vi "0-Write MDF.vi"(3 "List of Waypoints":T1 {"Waypoints Array"."Point Type" items=["Drive", "Round Port", "Round Starboard", "Stay"]}) -> ()   [LabVIEW 2011]
uses:
  0x2-OCU-Think Comm/0x2 Typedefs/ocuWaypoints.ctl
  0x2-OCU-Think Comm/0x2 Typedefs/ocuWaypoint.ctl
  0x2-OCU-Think Comm/0x2 Typedefs/waypointTypes.ctl
  2-Think/2 Typedefs/UTM Location.ctl
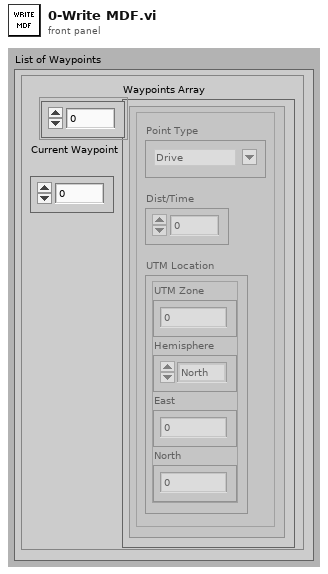
[diagram p1: front panel]
types:
  T1 = typedef "ocuWaypoints.ctl" = cluster{"Waypoints Array":T2[], "Current Waypoint":dbl}
  T2 = typedef "ocuWaypoint.ctl" = cluster{"Point Type":T3, "Dist/Time":dbl, "UTM Location":T4}
  T3 = typedef "waypointTypes.ctl" = u16
  T4 = typedef "UTM Location.ctl" = cluster{"UTM Zone":dbl, "Hemisphere":enum16{"North", "South"}, "East":dbl, "North":dbl}
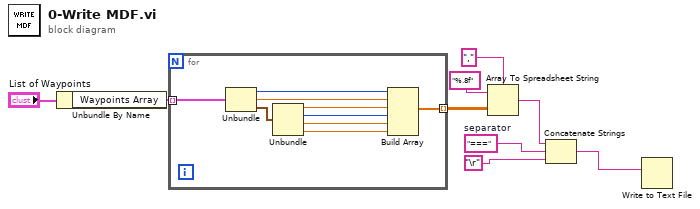
[diagram p0: block diagram]
diagram:
  w5 = "==="  # separator
  n1 = Unbundle By Name("List of Waypoints") -> ("Waypoints Array"=w2:T2[])
  n2 = for {
    tunnel: w2 -> [w18] mode=indexing
    tunnel: [w10] -> w1 mode=indexing
    n3 = Unbundle(w18) -> ("Point Type"=w16:T3, "Dist/Time"=w15:dbl, "UTM Location"=w17:T4)
    n4 = Unbundle(w17) -> ("UTM Zone"=w14:dbl, "Hemisphere"=w13:enum16{"North", "South"}, "East"=w12:dbl, "North"=w11:dbl)
    n5 = Build Array(w16, w15, w14, w13, w12, w11) -> (w10:dbl[])
  }
  n6 = Array To Spreadsheet String(delimiter (Tab)=",", array=w1, 3:"%.8f" ("format string")) -> (spreadsheet string=w7:string)
  n7 = Concatenate Strings(w7, w5, "\r") -> (w6:string)
  n8 = Write to Text File(text=w6) -> ()  [unwired: 3 in, 3 out]
